vi "Calculate F(x)_solution.vi"() -> (2 "val1":dbl, 3 "f(x)":dbl)   [LabVIEW 2023]
panel:
  out "Waveform Graph 2":dbl[](graph)
  out "Waveform Graph":dbl[](graph)
  out "Output Array":dbl[][](array[numeric])
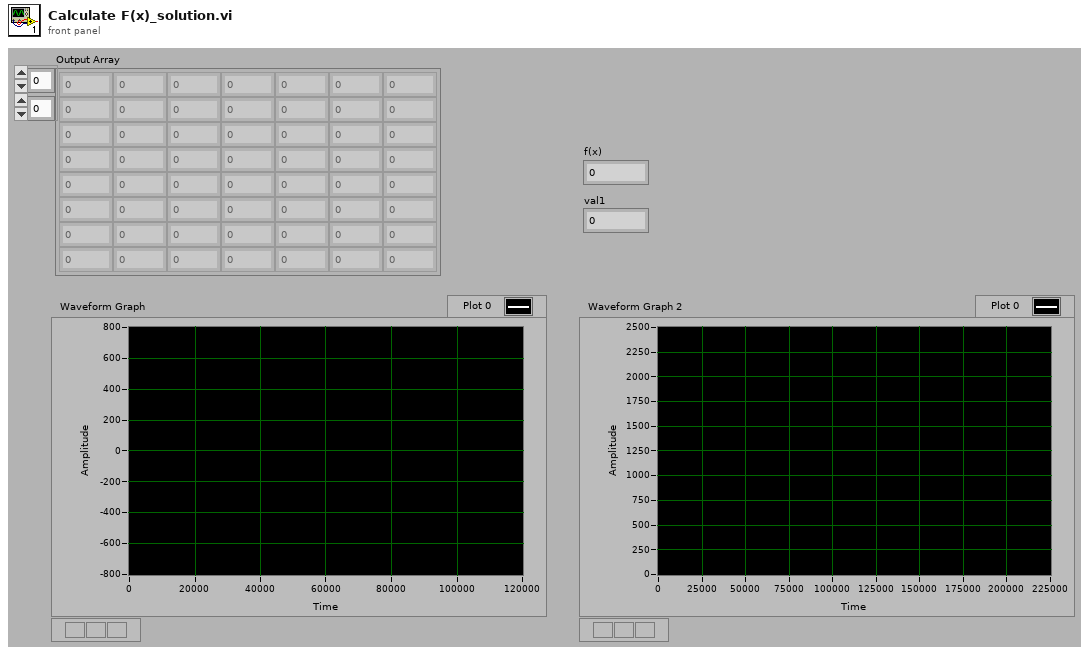
[diagram p1: front panel]
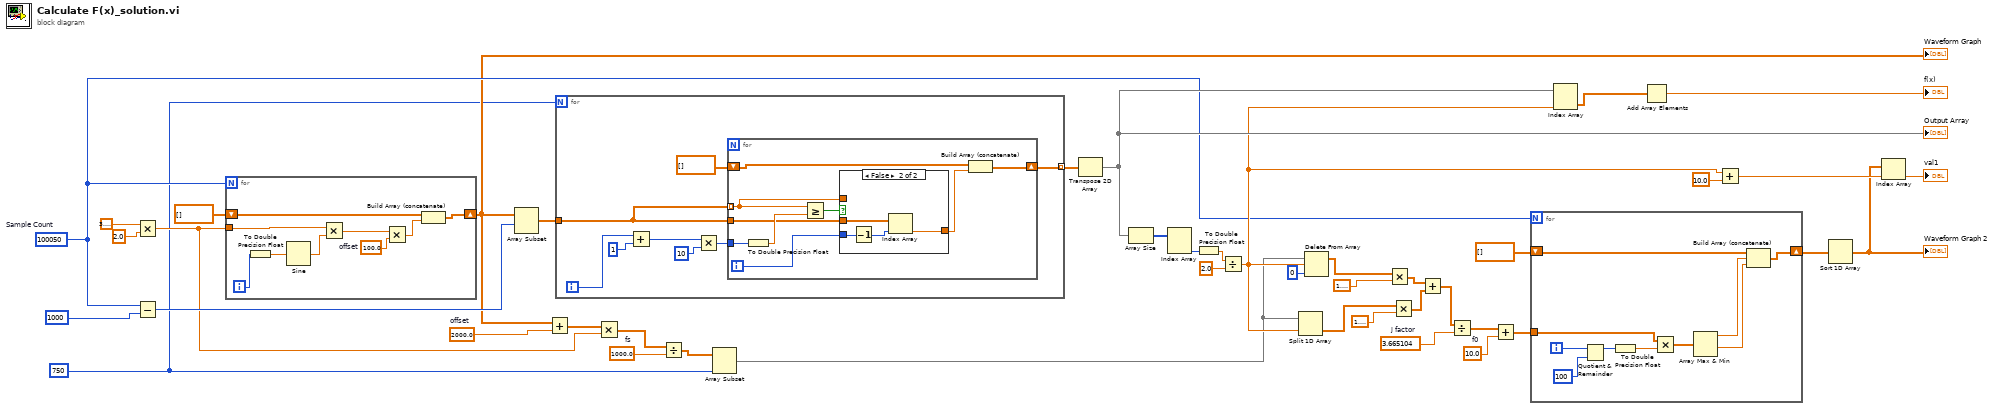
[diagram p0: block diagram]
diagram:
  w8 = 10.0  # f0
  w7 = 3.665104  # j factor
  w24 = 1000.0  # fs
  w22 = 2000.0  # offset
  w18 = 750 ("y")
  w28 = 100050  # Sample Count
  n1 = Multiply(x=3.141592653589793, y=2.0) -> (x*y=w20:dbl)
  n2 = Subtract(x=w28, y=1000) -> (x-y=w27:i32)
  n3 = for {
    N: w28 -> [_]
    shift-right: [w48] -> w21
    shift-left: dbl[] [] -> [w45]
    tunnel: w20 -> [w49]
    i -> [w52]
    w47 = 100.0  # offset
    n4 = To Double Precision Float(number=w52) -> (double precision float=w46:dbl)
    n5 = Sine(x=w46) -> (sin(x)=w51:dbl)
    n6 = Multiply(x=w49, y=w51) -> (x*y=w50:dbl)
    n7 = Multiply(x=w50, y=w47) -> (x*y=w44:dbl)
    n8 = Build Array (concatenate)(w45, w44) -> (w48:dbl[])
  }
  "Waveform Graph" <- w21
  n9 = Array Subset(array=w21, index=w27) -> (w26:dbl[])  [unwired: 1 in]
  n10 = Add(x=w21, y=w22) -> (x+y=w25:dbl[])
  n11 = for {
    N: w18 -> [_]
    tunnel: [w59] -> w43 mode=indexing
    tunnel: w26 -> [w54]
    i -> [w53]
    n12 = Add(x=w53, y=1) -> (x+y=w57:i32)
    n13 = Multiply(x=w57, y=10) -> (x*y=w55:i32)
    n14 = for {
      tunnel: w54 -> [w64] mode=indexing
      shift-right: [w63] -> w59
      shift-left: dbl[] [] ("array") -> [w61]
      tunnel: w55 -> [w69]
      tunnel: w54 -> [w65]
      i -> [w68]
      n15 = To Double Precision Float(number=w69) -> (double precision float=w66:dbl)
      n16 = Greater Or Equal?(x=w64, y=w66) -> (x >= y?=w67:bool)
      n17 = case shown="False" w67 {
        tunnel: w65 -> [_ w74]
        tunnel: w68 -> [_ w72]
        tunnel: [w70 w73] -> w62
        tunnel: w64 -> [w70 _]
        frame True {
        }
        frame False {
          n18 = Decrement(x=w72) -> (x-1=w71:i32)
          n19 = Index Array(array=w74, index=w71) -> (element=w73:dbl)
        }
      }
      n20 = Build Array (concatenate)(w61, w62) -> (w63:dbl[])
    }
  }
  n21 = Multiply(x=w25, y=w20) -> (x*y=w23:dbl[])
  n22 = Divide(x=w23, y=w24) -> (x/y=w19:dbl[])
  n23 = Array Subset(array=w19, length=w18) -> (w10:dbl[])  [unwired: 1 in]
  n24 = Transpose 2D Array(2D array=w43) -> (transposed array=w34:dbl[][])
  "Output Array" <- w34
  n25 = Array Size(array=w34) -> (size(s)=w42:i32[])
  n26 = Index Array(array=w42) -> (element #2=w40:i32)  [unwired: 2 in, 1 out]
  n27 = To Double Precision Float(number=w40) -> (double precision float=w1:dbl)
  n28 = Divide(x=w1, y=2.0) -> (x/y=w33:dbl)
  n29 = Split 1D Array(array=w10, index=w33) -> (second subarray=w12:dbl[])  [unwired: 1 out]
  n30 = Delete From Array(array=w10, length=w33, index=0) -> (array with subset deleted=w14:dbl[])  [unwired: 1 out]
  n31 = Multiply(x=w14, y=1.5707963267948966) -> (x*y=w15:dbl[])
  n32 = Multiply(x=w12, y=1.5707963267948966) -> (x*y=w16:dbl[])
  n33 = Add(x=w15, y=w16) -> (x+y=w17:dbl[])
  n34 = Divide(x=w17, y=w7) -> (x/y=w13:dbl[])
  n35 = Add(x=w13, y=w8) -> (x+y=w5:dbl[])
  n36 = for {
    N: w28 -> [_]
    shift-right: [w80] -> w38
    shift-left: dbl[] [] -> [w79]
    tunnel: w5 -> [w78]
    i -> [w84]
    n37 = Quotient & Remainder(x=w84, y=100) -> (x-y*floor(x/y)=w82:i32)  [unwired: 1 out]
    n38 = To Double Precision Float(number=w82) -> (double precision float=w75:dbl)
    n39 = Multiply(x=w78, y=w75) -> (x*y=w81:dbl[])
    n40 = Array Max & Min(array=w81) -> (max value=w77:dbl, min value=w76:dbl)  [unwired: 2 out]
    n41 = Build Array (concatenate)(w79, w77, w76) -> (w80:dbl[])
  }
  n42 = Index Array(array=w34, index (col)=w33) -> (element=w4:dbl[])  [unwired: 1 in]
  n43 = Add Array Elements(numeric array=w4) -> (sum=→"f(x)":dbl)
  n44 = Add(x=w33, y=10.0) -> (x+y=w35:dbl)
  n45 = Sort 1D Array(array=w38) -> (sorted array=w2:dbl[])
  "Waveform Graph 2" <- w2
  n46 = Index Array(array=w2, index=w35) -> (element=→"val1":dbl)
